vi "User Input.vi"() -> ()   [LabVIEW 2014]
doc: "This example shows how to use the User Input API VI for a console application. Prompts a user for input from stdin. The optional prompt parameter provides a prompt message without requiring a separate print command. This example will print: \"Input Name: \" and wait for the user input. Then it will bundle the \"Hello, \" string with the user input and output it to the String control."
uses:
  Console.lvlib
panel:
  out "String":string
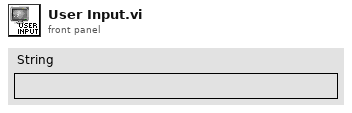
[diagram p1: front panel]
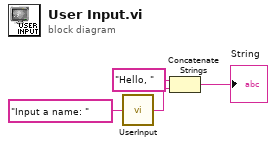
[diagram p0: block diagram]
diagram:
  n1 = call "UserInput.vi"("prompt"="Input a name: ") -> ("user input"=w2:string)
  n2 = Concatenate Strings("Hello, " ("string"), w2) -> (→"String":string)
